vi "CalStruct_Read.vi"(8 "error in":errorcluster) -> (0 "error out":errorcluster, 3 "Return Code":i32)   [LabVIEW 2015]
doc: "This function will read the calibration data from the DSP and place the information into the Calibration structure stored locally in the DLL."
uses:
  ScannerDiagDLL.dll
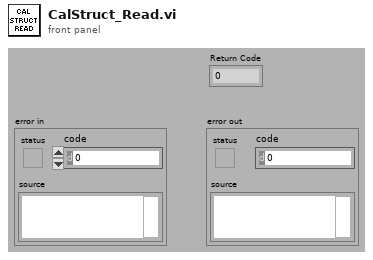
[diagram p1: front panel]
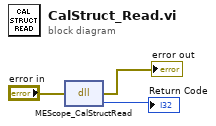
[diagram p0: block diagram]
diagram:
  n1 = dll-call lib="C:/SNAPON/ModisEdge/TabletScope/Test Sequence/Code Modules/DLL/ScannerDiagDLL.dll" fn="MEScope_CalStructRead"(error in="error in") -> (error out=→"error out":errorcluster, "return type"=→"Return Code":i32)  [unwired: 2 in, 1 out]
